vi "manual test deploy tool.vi"() -> ()   [LabVIEW 2013, in "configuration tests.lvlib"]
uses:
  configuration tests.lvlib
  Framework Configuration Classes/target configuration/PL_Target Configuration.lvclass
  Configuration Editor/subVIs/deployment configuration.ctl
  Configuration Editor/Classes/TBM Configuration Node/deployment configuration.ctl
  <vilib>/NI/Tag Bus Module Framework/root configuration/Target Types.ctl
  Framework Configuration Classes/target configuration/PL_Target Configuration.lvclass/PL_Target Configuration.ctl
  Framework Configuration Classes/target configuration/Write name.vi
  Framework Configuration Classes/target configuration/Write hostname.vi
  Framework Configuration Classes/target configuration/Write OS.vi
  Configuration Editor/PL Framework Configuration Tool.lvlib
  Configuration Editor/Classes/TBM Configuration Node/TBM Configuration Node.lvclass
  <vilib>/NI/Tag Bus Module Framework/root configuration/TBM configuration.lvclass
panel:
  out "error out":errorcluster
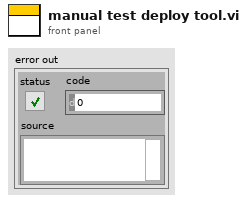
[diagram p1: front panel]
types:
  T1 = typedef "TBM configuration.lvclass/Target Types.ctl" = enum16{"Windows", "Mac", "Linux", "Linux RT ARM", "VxWorks", "Pharlap", "Other", "Linux RT x64"}
  T2 = typedef "PL Framework Configuration Tool.lvlib/TBM Configuration Node.lvclass/deployment configuration.ctl" = cluster{"local path":path, "remote path (relative to root)":path}
  T3 = typedef "PL Framework Configuration Tool.lvlib/deployment configuration.ctl" = cluster{"Target Configuration":refnum<class "PL_Target Configuration.lvclass">, "files":T2[]}
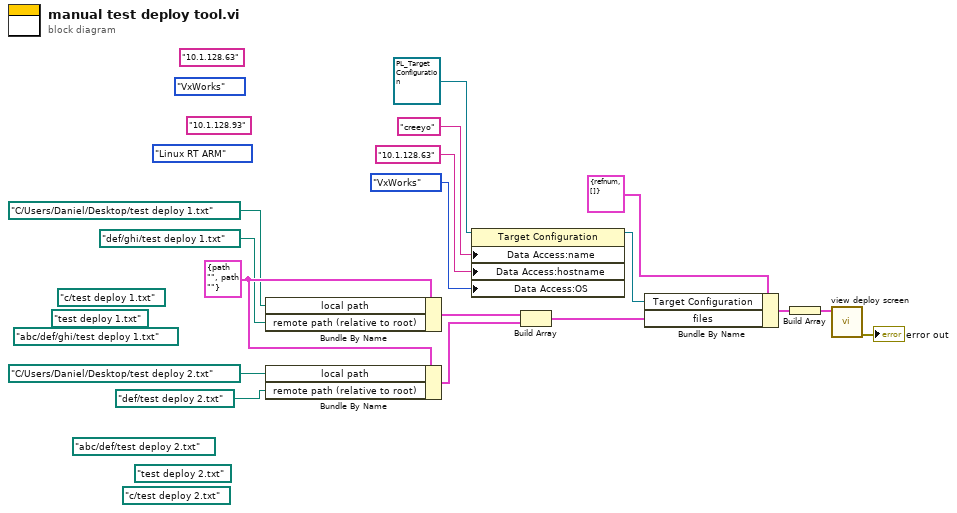
[diagram p0: block diagram]
diagram:
  (unwired) path "abc/def/test deploy 2.txt" ("remote path (relative to root)")
  (unwired) path "abc/def/ghi/test deploy 1.txt" ("remote path (relative to root)")
  (unwired) Target_Types."VxWorks" ("OS")
  (unwired) "10.1.128.63" ("hostname")
  (unwired) path "test deploy 1.txt" ("remote path (relative to root)")
  (unwired) path "c/test deploy 1.txt" ("remote path (relative to root)")
  (unwired) path "c/test deploy 2.txt" ("remote path (relative to root)")
  (unwired) Target_Types."Linux RT ARM" ("OS")
  (unwired) "10.1.128.93" ("hostname")
  (unwired) path "test deploy 2.txt" ("remote path (relative to root)")
  w9 = T2 {"local path"=path "", "remote path (relative to root)"=path ""} ("deployment configuration")
  n1 = Bundle By Name(cluster=w9, "local path"=path "C:/Users/Daniel/Desktop/test deploy 1.txt", "remote path (relative to root)"=path "def/ghi/test deploy 1.txt") -> (w3:T2)
  n2 = Bundle By Name(cluster=w9, "local path"=path "C:/Users/Daniel/Desktop/test deploy 2.txt", "remote path (relative to root)"=path "def/test deploy 2.txt") -> (w8:T2)
  n3 = property class="Target Configuration"(reference=refnum<class "PL_Target Configuration.lvclass"> refnum ("Target Configuration"), "Data Access:name"="creeyo" ("name"), "Data Access:hostname"="10.1.128.63" ("hostname"), "Data Access:OS"=Target_Types."VxWorks" ("OS")) -> (reference out=w12:refnum<class "PL_Target Configuration.lvclass">)  [unwired: 1 in, 1 out]
  n4 = Build Array(w3, w8) -> (w7:T2[])
  n5 = Bundle By Name(cluster=T3 {"Target Configuration"=refnum, "files"=[]}, "Target Configuration"=w12, "files"=w7) -> (w15:T3)
  n6 = Build Array(w15) -> (w14:T3[])
  n7 = call "view deploy screen.vi"("deployment configuration"=w14) -> ("error out"=→"error out":errorcluster)  [unwired: 10 in]
